vi "Top Level Calculator.vi"() -> ()   [LabVIEW 2014]
panel:
  out "Answer":dbl
  in  "y":dbl
  in  "x":dbl
  in  "Operator":T1(ring)
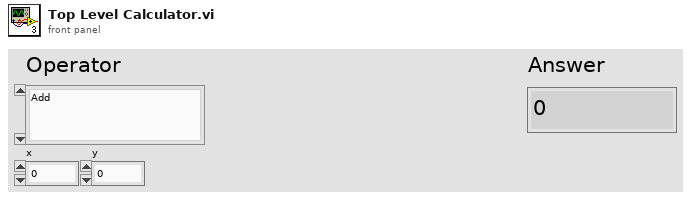
[diagram p1: front panel]
types:
  T1 = enum16{"Add", "Subtract", "Divide", "Multiply", "Power y^x"}
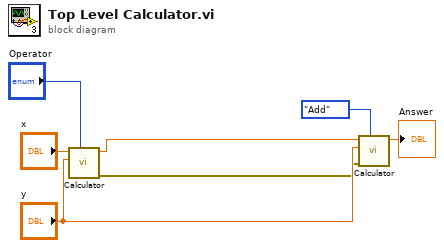
[diagram p0: block diagram]
diagram:
  n1 = call "Calculator.vi"("Operator"="Operator", "y"="y", "x"="x") -> ("error out"=w1:errorcluster, "Answer"=w5:dbl)  [unwired: 7 in]
  n2 = call "Calculator.vi"("Operator"=T1."Add", "error in (no error)"=w1, "y"="y", "x"=w5) -> ("Answer"=→"Answer":dbl)  [unwired: 6 in, 1 out]
